vi "Test Multipart String.vi"() -> ()   [LabVIEW 2020]
uses:
  HTTP Utils/Request/Request.lvclass
  lv-stream/stream/URI/URI.lvclass
  HTTP Utils/FormField/FormField.lvclass
  HTTP Utils/Method.ctl
  HTTP Utils/HTTP Utils.lvlib
panel:
  in  "String":string="POST /test HTTP/1.1\r\nHost: foo.example\r\nContent-Type: multipart/form-data;boundary=\"boundary\"\r\nContent-Length: 174\r\n\r\n--boundary\r\nContent-Disposition: form-data; name=\"field1\"\r\n\r\nvalue1\r\n--boundary\r\nContent-Disposition: form-data; name=\"field2\"; filename=\"example.txt\"\r\n\r\nvalue2\r\n--boundary--"
  out "Method":T1
  out "Target":string="/hello.htm"
  out "Version String":string="HTTP/1.1"
  out "Headers":cluster{"Header":string, "Value":string}[](array[cluster])=[{"Header"="accept-encoding", "Value"="gzip, deflate"}, {"Header"="accept-language", "Value"="en-us"}, {"Header"="connection", "Value"="Keep-Alive"}, {"Header"="host", "Value"="www.tutorialspoint.com"}, {"Header"="user-agent", "Value"="Mozilla/4.0 (compatible; MSIE5.01; Windows NT)"}]
  out "Is Form?":bool
  out "Form Fields":T2(array[cluster])
  # "Name"
  # "File"
  # "MIME/Type"
  # "Original Name"
  # "Temp Path"
  # "Value"
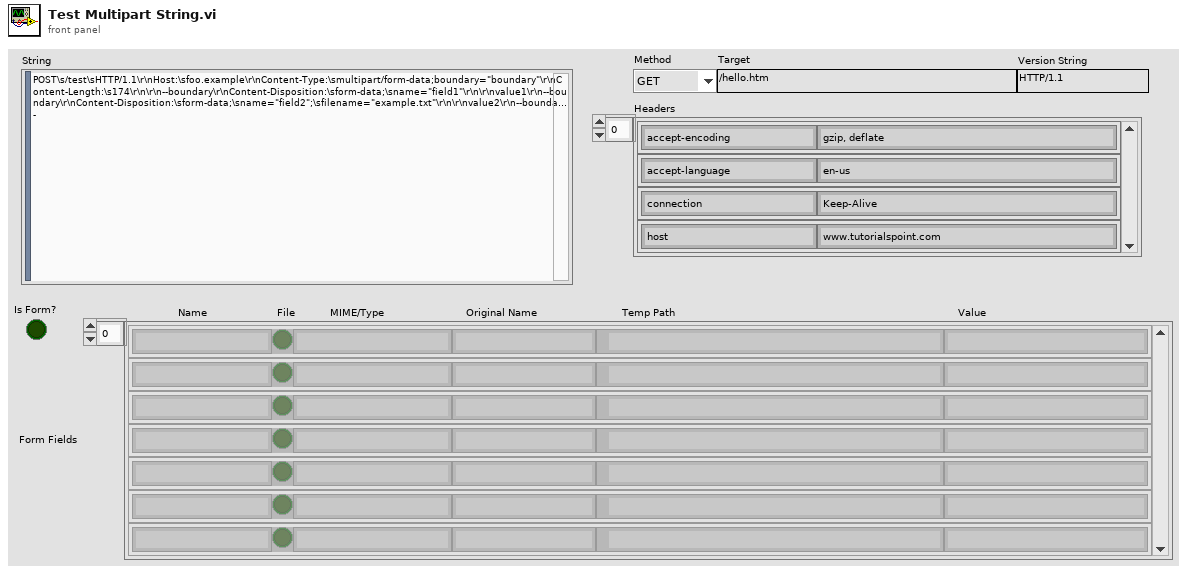
[diagram p1: front panel]
types:
  T1 = typedef "HTTP Utils.lvlib/Method.ctl" = enum16{"GET", "HEAD", "POST", "PUT", "DELETE", "CONNECT", "OPTIONS", "TRACE", "PATCH"}
  T2 = cluster{"Name":string, "Is File?":bool, "MIME Type":string, "Original Name":string, "Path":path, "Value":string}[]
  T3 = cluster{"Properties:Name":string, "Properties:Is File?":bool, "Properties:MIME Type":string, "Properties:Original Name":string, "Properties:Path":path, "Properties:Value":string}
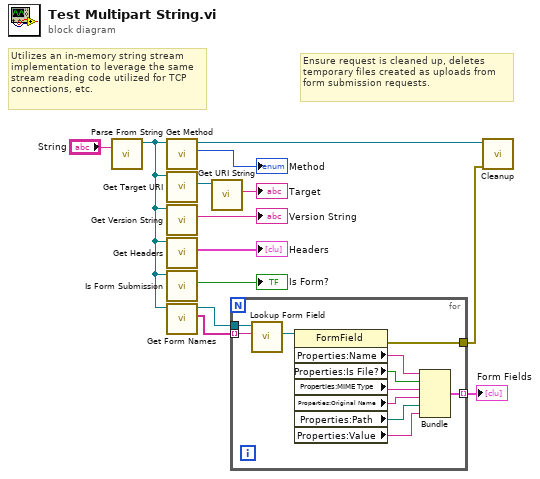
[diagram p0: block diagram]
diagram:
  # "Ensure request is cleaned up, deletes temporary files created as uploads from form submission requests."
  # "Utilizes an in-memory string stream implementation to leverage the same stream reading code utilized for TCP connections, etc."
  n1 = call "Parse From String.vi"("Request String"="String") -> ("Request out"=w3:refnum<class "Request.lvclass">)  [unwired: 9 in, 1 out]
  n2 = call "Get Method.vi"("Request in"=w3) -> ("Method"=→"Method":T1, "Request out"=w2:refnum<class "Request.lvclass">)  [unwired: 8 in, 1 out]
  n3 = call "Get Target URI.vi"("Request in"=w3) -> ("Target URI"=w12:refnum<class "URI.lvclass">)  [unwired: 8 in, 2 out]
  n4 = call "Get Version String.vi"("Request in"=w3) -> ("Version String"=→"Version String":string)  [unwired: 8 in, 2 out]
  n5 = call "Get Headers.vi"("Request in"=w3) -> ("Headers"=→"Headers":cluster{"Header":string, "Value":string}[])  [unwired: 8 in, 2 out]
  n6 = call "Is Form Submission.vi"("Request in"=w3) -> ("Is Form Submission?"=→"Is Form?":bool)  [unwired: 8 in, 2 out]
  n7 = call "Get Form Names.vi"("Request in"=w3) -> ("Form Names"=w6:string[], "Request out"=w4:refnum<class "Request.lvclass">)  [unwired: 8 in, 1 out]
  n8 = call "Get URI String.vi"("URI in"=w12) -> ("URI String"=→"Target":string)  [unwired: 8 in, 2 out]
  n9 = for {
    tunnel: w4 -> [w24]
    tunnel: w6 -> [w23] mode=indexing
    tunnel: [w15] -> w5 mode=indexing
    tunnel: [w14] -> w1
    n10 = call "Lookup Form Field.vi"("Name"=w23, "Request in"=w24) -> ("Field"=w22:refnum<class "FormField.lvclass">)  [unwired: 6 in, 3 out]
    n11 = property class="FormField"(reference=w22) -> (error out=w14:errorcluster, "Properties:Name"=w21:string, "Properties:Is File?"=w19:bool, "Properties:MIME Type"=w20:string, "Properties:Original Name"=w18:string, "Properties:Path"=w16:path, "Properties:Value"=w17:string)  [unwired: 1 in, 1 out]
    n12 = Bundle("Properties:Name"=w21, "Properties:Is File?"=w19, "Properties:MIME Type"=w20, "Properties:Original Name"=w18, "Properties:Path"=w16, "Properties:Value"=w17) -> (w15:T3)  [unwired: 1 in]
  }
  "Form Fields" <- w5
  n13 = call "Cleanup.vi"("error in (no error)"=w1, "Request in"=w2) -> ()  [unwired: 9 in, 1 out]
